vi "Test_Populate.vi"() -> ()   [LabVIEW 2019]
uses:
  ClassLoader.lvlib
panel:
  in  "Listbox":i32(listbox)
  in  "Sort Alphabetically instead of by Hierarchy?(T)":bool=TRUE
  in  "Ring":u16(ring) items=["Addressed Msg", "Batch End Msg", "Batch Msg", "Bypass Msg", "Close File Msg", "Cycle Msg", "Data Msg", "Data Tracker Msg", "Display Pop Up Msg", "Flex Msg", "Flush Sequncer Msg", "Instrument Handler Response Msg", "Instrument Msg", "Interrupt Sequncer Msg", "Last Ack", "Launch Subscriber Msg", "List Driver Aliases Msg", "List Instruments Msg", "Load and Run Sequence Msg", "Loop Msg", "Message", "Multi Instrument Batch Msg", "Multi Instrument Msg", "Nested Sequence Msg", "Open File Msg", "Ping Msg", "Publish Msg", "Publisher Msg", "Register Instrument Msg", "Reorder Driver Aliases Msg", "Response Msg", "Sender Msg", "Sequencer Msg", "Show Actor Msg", "Start Instrument Calibration Msg", "Stop Msg", "Sub Panel Insertion Msg", "Subscribe Msg", "Targetted Msg", "Timed Msg", "Unsubscribe Msg", "Wait Msg"]
  in  "Pre-Clear Tree?(T)":bool=TRUE
  in  "Hierarchy Filter(empty=all)":string
  in  "Close Reference?(T)":bool=TRUE
  in  "Tree":string(tree)
  out "Success?":bool
  out "error out":errorcluster
  in  "error in (no error)":errorcluster
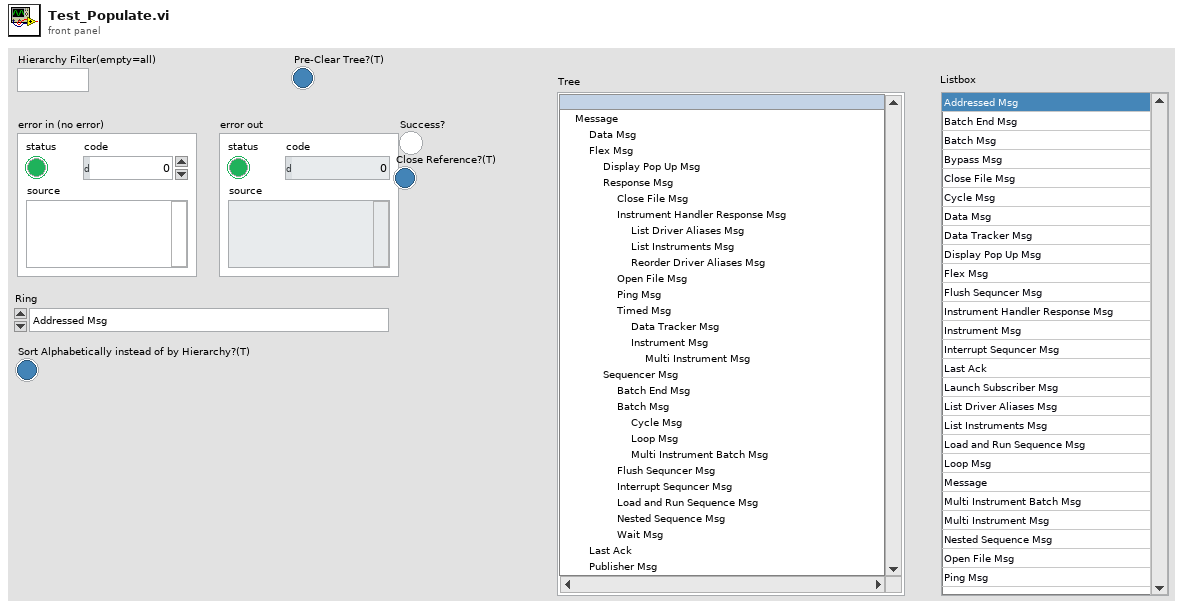
[diagram p1: front panel]
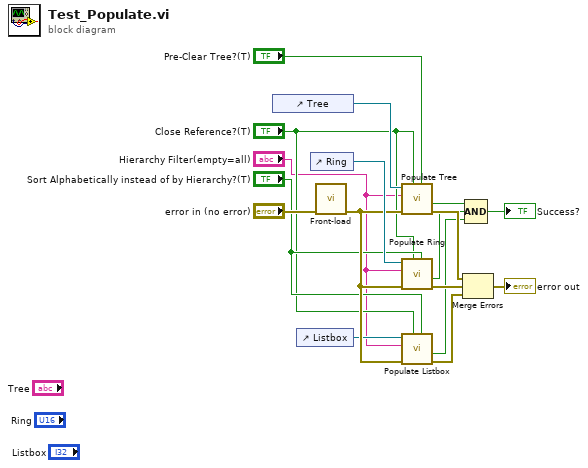
[diagram p0: block diagram]
diagram:
  n1 = control-ref of="Tree"() -> (w16:refnum<vi>)
  n2 = control-ref of="Listbox"() -> (w5:refnum<vi>)
  n3 = control-ref of="Ring"() -> (w12:refnum<vi>)
  n4 = call "Front-load.vi"("error in (no error)"="error in (no error)") -> ("error out"=w7:errorcluster)  [unwired: 9 in, 1 out]
  n5 = call "Populate Tree.vi"("Pre-Clear Tree?(T)"="Pre-Clear Tree?(T)", "Close Reference?(T)"="Close Reference?(T)", "error in (no error)"=w7, "Hierarchy Filter(empty=all)"="Hierarchy Filter(empty=all)", "TreeControl in"=w16) -> ("error out"=w15:errorcluster, "Success?"=w14:bool)  [unwired: 4 in, 1 out]
  n6 = call "Populate Ring.vi"("Sort Alphabetically instead of by Hierarchy?(T)"="Sort Alphabetically instead of by Hierarchy?(T)", "Close Reference?(T)"="Close Reference?(T)", "error in (no error)"=w7, "Hierarchy Filter(empty=all)"="Hierarchy Filter(empty=all)", "Ring in"=w12) -> ("error out"=w10:errorcluster, "Success?"=w8:bool)  [unwired: 4 in, 1 out]
  n7 = call "Populate Listbox.vi"("Sort Alphabetically instead of by Hierarchy?(T)"="Sort Alphabetically instead of by Hierarchy?(T)", "Close Reference?(T)"="Close Reference?(T)", "error in (no error)"=w7, "Hierarchy Filter(empty=all)"="Hierarchy Filter(empty=all)", "ListBox in"=w5) -> ("error out"=w6:errorcluster, "Success?"=w1:bool)  [unwired: 4 in, 1 out]
  n8 = Merge Errors(w15, w10, w6) -> (→"error out":errorcluster)
  n9 = Compound Arithmetic op=AND(w14, w8, w1) -> (→"Success?":bool)
